vi "Send Algorithm Result User Event_RC.vi"(7 "Message Priority (Normal)":T3=enum."Normal", 8 "error in (no error)":errorcluster, 10 "Algorithm Result Data":T1, 11 "Message Enqueuer":refnum<class "Message Enqueuer.lvclass">) -> (0 "error out":errorcluster, 3 "Message Enqueuer out":refnum<class "Message Enqueuer.lvclass">)   [LabVIEW 2019, in "Algorithm Result User Event_RC Msg.lvclass"]
doc: "This VI sends the message to an actor."
uses:
  Algorithm Result User Event_RC Msg.lvclass
  <vilib>/ActorFramework/Message Enqueuer/Message Enqueuer.lvclass
  C:/Program Files/National Instruments/LabVIEW 2019/vi.lib/ActorFramework/Message/Message.lvclass
  <vilib>/ActorFramework/Message Enqueuer/Message Priority.ctl
  <vilib>/vision/Image Controls.llb/IMAQ Image.ctl
  Controls/Result Cluster_RC.ctl
  Rack Controller.lvclass
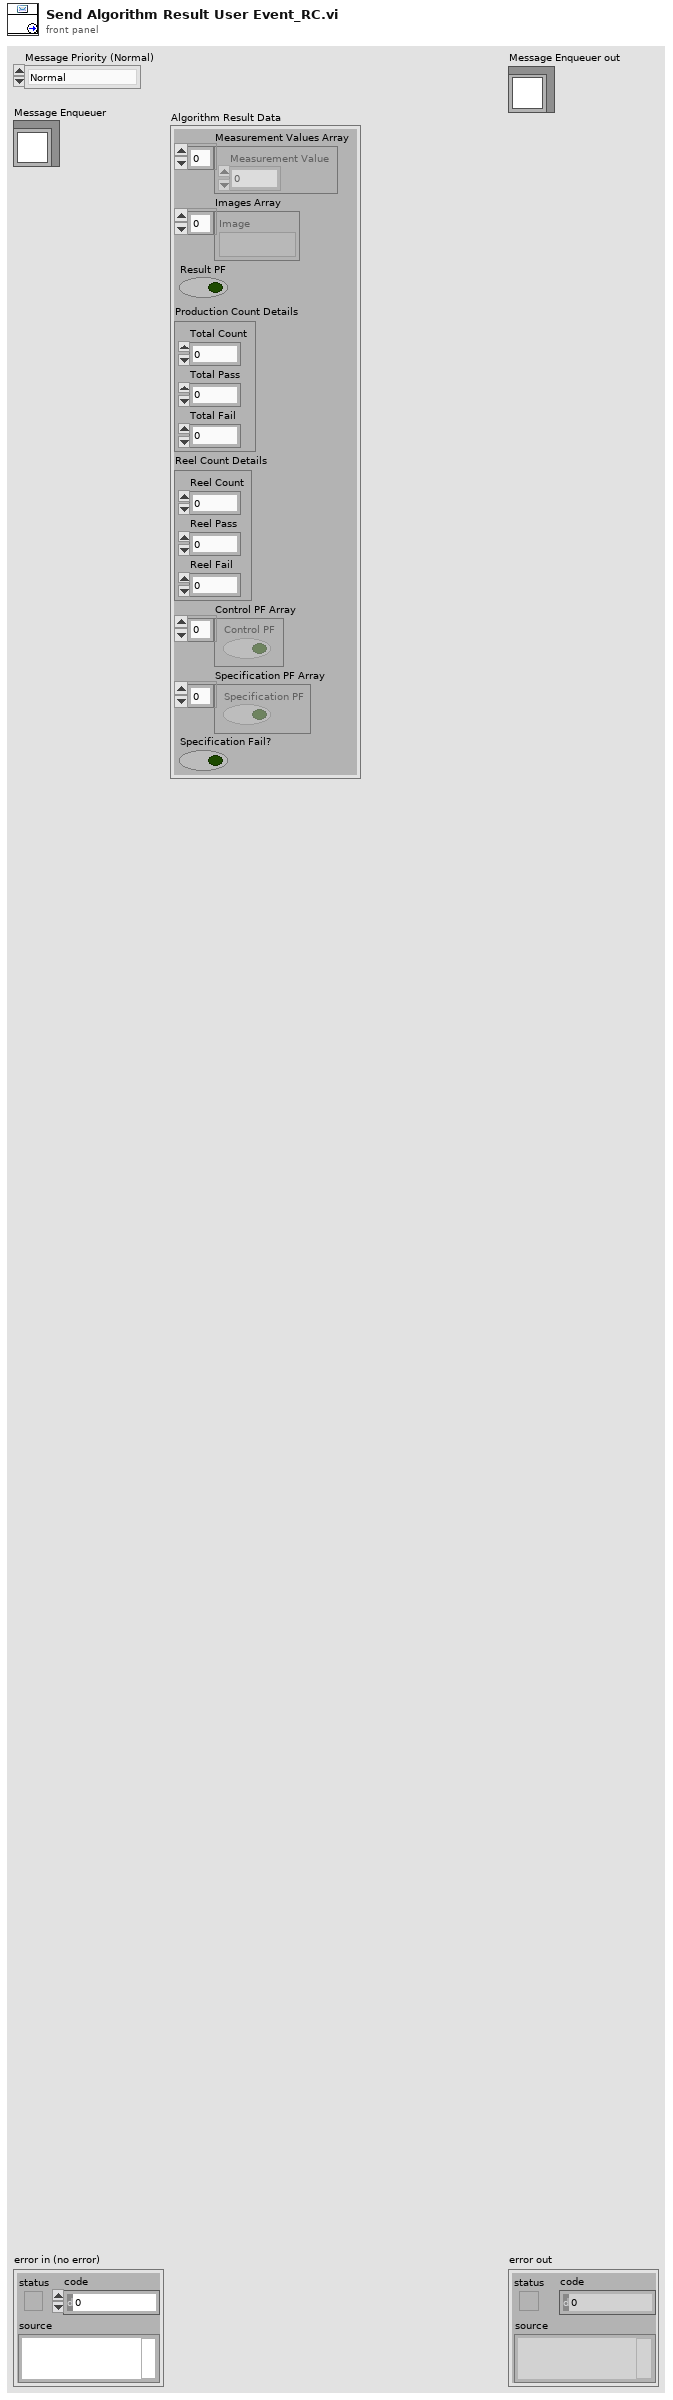
[diagram p1: front panel]
types:
  T1 = typedef "Rack Controller.lvclass/Result Cluster_RC.ctl" = cluster{"Measurement Values Array ":dbl[], "Images Array":T2[], "Result PF":bool, "Production Count Details":cluster{"Total Fail":u64, "Total Pass":u64, "Total Count":u64}, "Reel Count Details":cluster{"Reel Fail":u64, "Reel Pass":u64, "Reel Count":u64}, "Control PF Array":bool[], "Specification PF Array":bool[], "Specification Fail?":bool}
  T2 = typedef "IMAQ Image.ctl" = refnum<image>
  T3 = typedef "Actor Framework.lvlib/Message Enqueuer.lvclass/Message Priority.ctl" = enum16{"Low", "Normal", "High"}
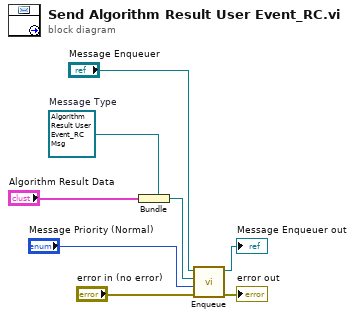
[diagram p0: block diagram]
diagram:
  w5 = refnum<class "Algorithm Result User Event_RC Msg.lvclass"> refnum  # Message Type
  n1 = Bundle(cluster=w5, "Algorithm Result Data") -> (w4:refnum<class "Algorithm Result User Event_RC Msg.lvclass">)
  n2 = call <vilib>:"Enqueue.vi"("error in (no error)"="error in (no error)", "Message Priority (Normal)"="Message Priority (Normal)", "Message"=w4, "Message Enqueuer in"="Message Enqueuer") -> ("error out"=→"error out":errorcluster, "Message Enqueuer out"=→"Message Enqueuer out":refnum<class "Message Enqueuer.lvclass">)  [unwired: 6 in]
